vi "readLaser.vi"(8 "error in":errorcluster) -> (2 "Cm":u16)   [LabVIEW 2018]
uses:
  <vilib>/Studica/Studica Toolkit/Background/I2C Channel.ctl
panel:
  out "error out 5":errorcluster
  out "error out 4":errorcluster
  out "error out 3":errorcluster
  out "error out 2":errorcluster
  out "error out":errorcluster
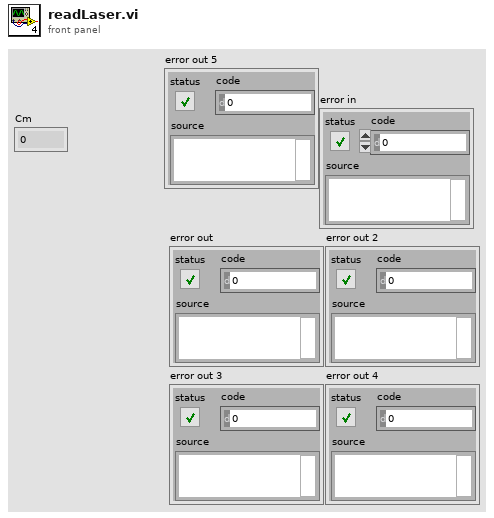
[diagram p1: front panel]
types:
  T1 = typedef "I2C Channel.ctl" = enum16{"Not Connected", "A", "B"}
  T2 = cluster{"I2C Channel":T1, "FPGA VI Reference Out":refnum<k20>}
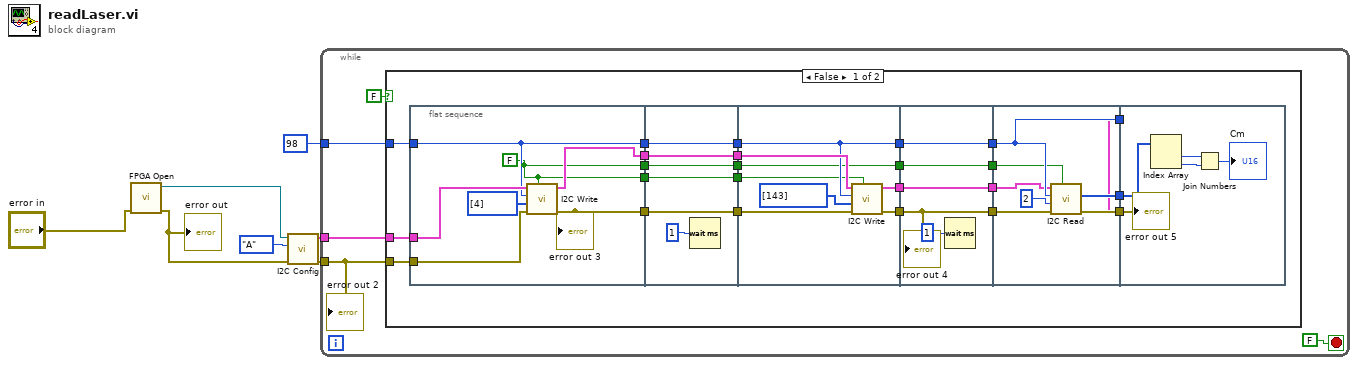
[diagram p0: block diagram]
diagram:
  n1 = call <vilib>:"FPGA Open.vi"("error in (no error)"="error in") -> ("error out"=w1:errorcluster, "FPGA Reference Out"=w3:refnum<k20>)  [unwired: 9 in]
  "error out" <- w1
  n2 = call <vilib>:"I2C Config.vi"("error in (no error)"=w1, "I2C Channel"=I2C_Channel."A", "FPGA Reference"=w3) -> ("error out"=w4:errorcluster, "I2C Ref Out"=w5:T2)  [unwired: 7 in]
  n3 = while {
    tunnel: u8 98 -> [w11]
    tunnel: w5 -> [w9]
    tunnel: w4 -> [w8]
    stop <- FALSE stop-if-true
    n4 = case shown="False" FALSE {
      tunnel: w11 -> [w37 _]
      tunnel: w9 -> [w21 _]
      tunnel: w8 -> [w19 _]
      frame False {
        n5 = flat-sequence {
          tunnel: w21 -> [w44]
          tunnel: w37 -> [w43]
          tunnel: [w41] -> w36
          tunnel: [w43] -> w33
          tunnel: [w42] -> w20
          tunnel: w19 -> [w40]
          tunnel: [w39] -> w18
          tunnel: [w39] -> w16
          tunnel: w36 -> [w49]
          tunnel: [w49] -> w35
          tunnel: [w48] -> w34
          tunnel: w33 -> [w47]
          tunnel: [w47] -> w32
          tunnel: w20 -> [w48]
          tunnel: w18 -> [w46]
          tunnel: [w46] -> w17
          tunnel: w16 -> [w45]
          tunnel: [w45] -> w15
          tunnel: w35 -> [w58]
          tunnel: w34 -> [w55]
          tunnel: w32 -> [w56]
          tunnel: [w53] -> w31
          tunnel: [w54] -> w29
          tunnel: [w56] -> w27
          tunnel: w17 -> [w52]
          tunnel: w15 -> [w51]
          tunnel: [w51] -> w14
          tunnel: w31 -> [w62]
          tunnel: [w62] -> w30
          tunnel: w29 -> [w61]
          tunnel: [w61] -> w28
          tunnel: w27 -> [w60]
          tunnel: [w60] -> w26
          tunnel: w14 -> [w59]
          tunnel: [w59] -> w13
          tunnel: w30 -> [w67]
          tunnel: w28 -> [w71]
          tunnel: w26 -> [w70]
          tunnel: [w65] -> w25
          tunnel: [w66] -> w24
          tunnel: [w70] -> w23
          tunnel: [w68] -> w22
          tunnel: w13 -> [w64]
          tunnel: w25 -> [_]
          tunnel: w24 -> [w72]
          tunnel: w23 -> [_]
          tunnel: w22 -> [w76]
          frame #0 {
            w39 = FALSE ("Keep Bus Busy")
            n6 = call <vilib>:"I2C Write.vi"("Keep Bus Busy"=w39, "error in (no error)"=w40, "Data to Write"=u8[] [4], "Slave Address (7-bit)"=w43, "I2C Ref In"=w44) -> ("error out"=w42:errorcluster, "I2C Ref Out"=w41:T2)  [unwired: 5 in]
            "error out 3" <- w42
          }
          frame #1 {
            n7 = Wait (ms)(milliseconds to wait=u32 1) -> ()  [unwired: 1 out]
          }
          frame #2 {
            n8 = call <vilib>:"I2C Write.vi"("Keep Bus Busy"=w52, "error in (no error)"=w55, "Data to Write"=u8[] [143], "Slave Address (7-bit)"=w56, "I2C Ref In"=w58) -> ("error out"=w54:errorcluster, "I2C Ref Out"=w53:T2)  [unwired: 5 in]
          }
          frame #3 {
            n9 = Wait (ms)(milliseconds to wait=u32 1) -> ()  [unwired: 1 out]
            "error out 4" <- w61
          }
          frame #4 {
            n10 = call <vilib>:"I2C Read.vi"("Keep Bus Busy"=w64, "error in (no error)"=w71, "Bytes to Read"=u32 2 ("Byte Count"), "Slave Address (7-bit)"=w70, "I2C Ref In"=w67) -> ("error out"=w66:errorcluster, "Data Out"=w68:u8[], "I2C Ref Out"=w65:T2)  [unwired: 4 in]
          }
          frame #5 {
            n11 = Index Array(array=w76) -> (element #1=w75:u8, element #2=w74:u8)  [unwired: 2 in]
            n12 = Join Numbers(hi=w75, lo=w74) -> ((hi.lo)=→"Cm":u16)
            "error out 5" <- w72
          }
        }
      }
      frame True {
      }
    }
    "error out 2" <- w8
  }
